vi "Check Component Settings Change.vi"(8 "error in (no error)":errorcluster, 10 "new component settings":T1[](array[typedef]), 11 "current component settings":T1[](array[typedef])) -> (0 "error out":errorcluster, 2 "new component settings dup":T1[](array[typedef]), 3 "changed?":bool)   [LabVIEW 2020, in "DSF System Explorer.lvlib"]
uses:
  DSF System Explorer.lvlib
  DSF Core.lvlibp/Typedefs/DSF Settings Info.ctl
  Source/DSF Core.lvlibp
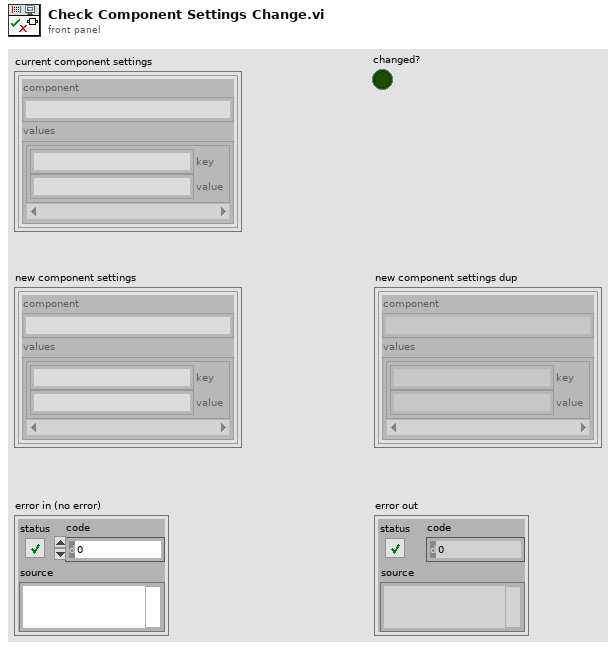
[diagram p1: front panel]
types:
  T1 = typedef "DSF Core.lvlibp/DSF Settings Info.ctl" = cluster{"component":string, "values":cluster{"key":string, "value":string}[]}
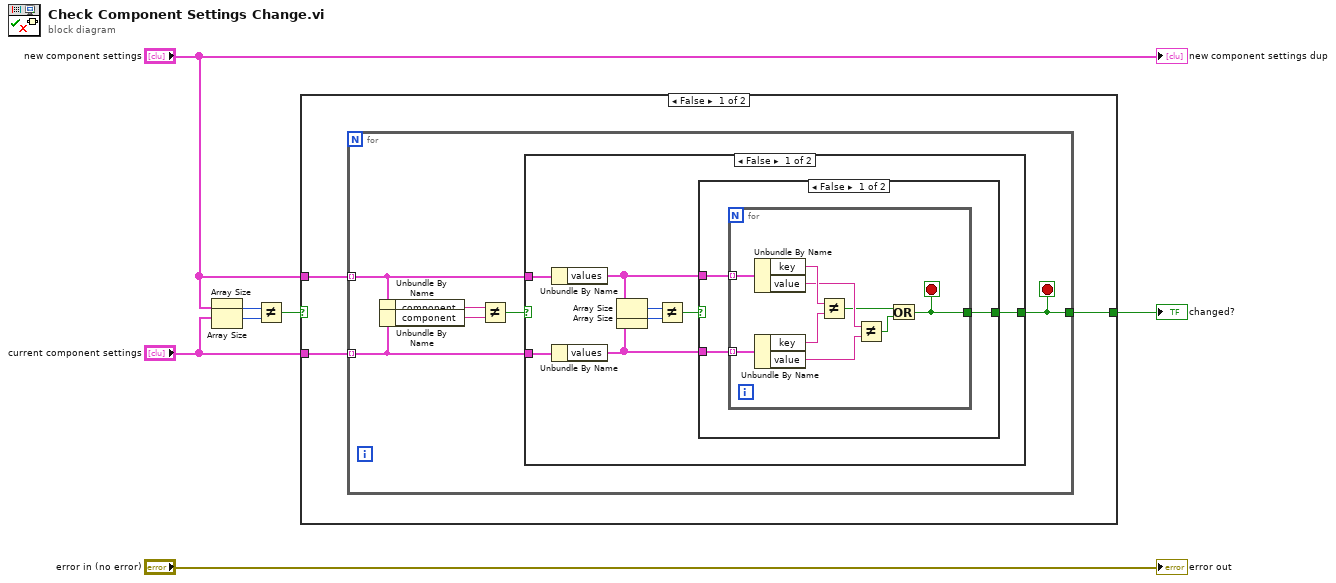
[diagram p0: block diagram]
diagram:
  n1 = Array Size(array="new component settings") -> (size(s)=w6:i32)
  n2 = Array Size(array="current component settings") -> (size(s)=w7:i32)
  n3 = Not Equal?(x=w6, y=w7) -> (x != y?=w5:bool)
  n4 = case shown="False" w5 {
    selector: w5 -> [_ w39]
    tunnel: [w8 w39] -> w4
    tunnel: "new component settings" -> [w9 _]
    tunnel: "current component settings" -> [w10 _]
    frame False {
      n5 = for {
        tunnel: w10 -> [w11] mode=indexing
        tunnel: w9 -> [w12] mode=indexing
        tunnel: [w13] -> w8
        stop <- w13 stop-if-true
        n6 = Unbundle By Name(w12) -> ("component"=w15:string)
        n7 = Unbundle By Name(w11) -> ("component"=w16:string)
        n8 = Not Equal?(x=w15, y=w16) -> (x != y?=w14:bool)
        n9 = case shown="False" w14 {
          selector: w14 -> [_ w38]
          tunnel: [w17 w38] -> w13
          tunnel: w12 -> [w23 _]
          tunnel: w11 -> [w24 _]
          frame False {
            n10 = Unbundle By Name(w23) -> ("values"=w20:cluster{"key":string, "value":string}[])
            n11 = Unbundle By Name(w24) -> ("values"=w19:cluster{"key":string, "value":string}[])
            n12 = Array Size(array=w20) -> (size(s)=w21:i32)
            n13 = Array Size(array=w19) -> (size(s)=w22:i32)
            n14 = Not Equal?(x=w21, y=w22) -> (x != y?=w18:bool)
            n15 = case shown="False" w18 {
              selector: w18 -> [_ w37]
              tunnel: w20 -> [w27 _]
              tunnel: w19 -> [w26 _]
              tunnel: [w25 w37] -> w17
              frame False {
                n16 = for {
                  tunnel: w27 -> [w36] mode=indexing
                  tunnel: w26 -> [w35] mode=indexing
                  tunnel: [w28] -> w25
                  stop <- w28 stop-if-true
                  n17 = Unbundle By Name(w36) -> ("key"=w34:string, "value"=w31:string)
                  n18 = Unbundle By Name(w35) -> ("key"=w33:string, "value"=w32:string)
                  n19 = Not Equal?(x=w34, y=w33) -> (x != y?=w29:bool)
                  n20 = Not Equal?(x=w31, y=w32) -> (x != y?=w30:bool)
                  n21 = Or(x=w29, y=w30) -> (x .or. y?=w28:bool)
                }
              }
              frame True {
              }
            }
          }
          frame True {
          }
        }
      }
    }
    frame True {
    }
  }
  "changed?" <- w4
  "new component settings dup" <- "new component settings"
  "error out" <- "error in (no error)"
